vi "Lines GetSessionByName.vi"(8 "error in (no error)":errorcluster, 10 "[] Session Name":string, 11 "Config Text List":string[](array[string])=["[Datalog_Path]", "datalog_name_rule_1={Customer_ID}/{Device_Name}/{Customer_LotNo}/{Sub_LotNo}/", "datalog_name_rule_2={Subcon}_{Tester_ID}_{Mode_Code}_{Device_Name}_{Program_Name}_{Customer_LotNo}_{Sub_LotNo}_{Test_BinNo}_{Test_Code}_{End_Time}", "[Datalog_Type]", "edl_flag = false", "stdf_flag = true", "gdf_flag = true", "summary_flag = true", "txt_flag = true", "stdfconvert_flag = true", "[PackTestResult]", "PackTestResult = true", "PackFileType = gz", "PackFileSet = S", "[INPUT_OI_tester_id]", "Name = Tester_ID", "Pattern = ^[A-Z]|[0-9]+\\S*$", "Index = 0", "[INPUT_OI_operator_id]", "Name = Operator_ID", "Pattern = ^[A-Z]|[0-9]+\\S*$", "Index = 1", "[INPUT_OI_device_name]", "Name = Device_Name", "Pattern = ^[A-Z]|[0-9]+\\S*$", "Index = 2", "[INPUT_OI_lot_no]", "Name = Customer_LotNo", "Pattern = ^[A-Z]|[0-9]+\\S*$", "Index = 3", "[INPUT_OI_sublot]", "Name = Sub_LotNo", "Pattern = ^[A-Z]+[0-9]+\\S*$", "Index = 4", "[INPUT_OI_mode_code]", "Name = Mode_Code", "Pattern = ^FT1$", "Index = 5", "[INPUT_OI_test_code]", "Name = Test_Code", "Pattern = ^R\\d+(\\.\\d+)?$", "Index = 6", "[INPUT_OI_test_bin_no]", "Name = Test_BinNo", "Pattern = ^ALL$", "Index = 7", "[TestCode_Config]", "R0=P1", "R0.1=P2", "R0.2=P3", "R0.3=P4", "R0.4=P5", "R0.5=P6", "R0.6=P7", "R0.7=P8", "R1=R1", "R1.1=R1.1", "R1.2=R1.2", "R2=R2", "R2.1=R2.1", "R2.2=R2.2", "R3=R3", "R3.1=R3.1", "R3.2=R3.2", "R4=R4", "R4.1=R4.1", "R4.2=R4.2", "R5=R5", "R5.1=R5.1", "R5.2=R5.2", "R6=R6", "R6.1=R6.1", "R6.2=R6.2", "Q0=Q0", "Q0.1=Q0.1", "Q1=Q1", "Q2=Q2", "Q3=Q3", "Q4=Q4", "Q5=Q5", "Q6=Q6", "Q7=Q7", "[Stdf_variable_Config]", "Mode_Code=TEST_COD", "Test_Code=FLOW_ID", "[Stdf_constant_Config]", "JCET=FACIL_ID", "25C=TST_TEMP", "[special Control Flag]", "tester_check_flag = 0", "application_mode_flag = 0", "exec_input_flag = 0", "databridge_flag = 0", "[efuse check condition]", "efuse_check_flag = 0", "T8980+T9980=T9900或S8980+S9980=S9900或H8980+H9980=H9900（具体要看每个产品以什么方式体现）", "T9980<10", "[HardBin_Pass]", "PASS_BIN=1,2", "[HardBin_alarm]", "1<95%", "2>0.5%", "[HardBin_Define]", "1=PASS", "2=openshort", "3=functionfail", "4=functionfail", "5=functionfail", "6=functionfail", "8=functionfail", "[SoftBin_Pass]", "PASS_BIN=101,102", "[SoftBin_alarm]", "201>0.5%", "301>0.2%", "[SoftBin_Define]", "1=PASS_CLASS1", "101=RC_PASS", "200=OS_DPS_Short_failed_200", "220=OS_Func_VSS_RPT1_failed_220", "221=OS_PPMU_VSS_failed_221", "310=DC_VIH_VDDH_failed_310", "311=DC_VIL_VDDL_failed_311", "312=DC_IIHL_failed_312", "330=DC_VOHL_failed_330", "340=FC_IOZ_Func_failed_340", "341=DC_IOZ_failed_341", "370=DC_IDDDQ_Func_failed_370", "371=DC_IDDDQ_failed_371", "400=FC_BSCAN_failed_400", "410=FC_MBIST_RAM_SLOW_failed_410", "411=FC_MBIST_ROM_BASIC_failed_411", "412=FC_MBIST_SLOW_INCR1_failed_412", "413=FC_MBIST_SLOW_INCR2_failed_413", "414=FC_MBIST_CPU_ALL_failed_414", "415=FC_MBIST_FEPHY_failed_415", "416=FC_MBIST_ROM_FEPHY_failed_416", "420=FC_CHAIN_LOW_failed_420", "430=FC_STUCK_LOW_R02_1_430", "431=FC_STUCK_LOW_R02_1_431", "432=FC_STUCK_LOW_R02_2_432", "433=FC_STUCK_LOW_R02_3_433", "434=FC_STUCK_LOW_R02_4_434", "435=FC_STUCK_LOW_R02_5_435", "436=FC_STUCK_LOW_R02_6_436", "437=FC_STUCK_LOW_R02_7_437", "440=FC_TRANS_LOW_R02_failed_440", "441=FC_TRANS_LOW_1_failed_441", "442=FC_TRANS_LOW_2_failed_442", "443=FC_TRANS_LOW_3_failed_443", "444=FC_TRANS_LOW_4_failed_444", "445=FC_TRANS_LOW_5_failed_445", "446=FC_TRANS_LOW_6_failed_446", "447=FC_TRANS_LOW_7_failed_447", "448=FC_TRANS_LOW_8_failed_448", "449=FC_TRANS_LOW_9_failed_449", "450=FC_TRANS_LOW_10_failed_450", "451=FC_TRANS_LOW_11_failed_451", "452=FC_TRANS_LOW_12_failed_452", "453=FC_TRANS_LOW_13_failed_453", "454=FC_TRANS_LOW_14_failed_454", "455=FC_TRANS_LOW_15_failed_455", "456=FC_TRANS_LOW_16_failed_456", "457=FC_TRANS_LOW_17_failed_457", "458=FC_TRANS_LOW_18_failed_458", "460=FC_TRANS_LOW_GPU_1_failed_460", "461=FC_TRANS_LOW_GPU_2_failed_461", "462=FC_TRANS_LOW_GPU_3_failed_462", "463=FC_TRANS_LOW_GPU_4_failed_463", "464=FC_TRANS_LOW_GPU_5_failed_464", "465=FC_TRANS_LOW_GPU_6_failed_465", "471=FC_TRANS_LOW_CPU_1_failed_471", "472=FC_TRANS_LOW_CPU_2_failed_472", "473=FC_TRANS_LOW_CPU_3_failed_473", "480=FC_TRANS_LOW_GPU_failed_480", "490=FC_TRANS_LOW_CPU_failed_490", "500=FC_MBIST_CPU_ALL_GB_failed_500", "501=FC_MBIST_CPU_ALL_0P94_GB_failed_501", "510=BIST_USB3_EXTLP_0P95_GB_failed_510", "511=BIST_USB3_INTLP_0P95_GB_failed_511", "520=BIST_USB3_ASYNC_failed_520", "600=BIST_DDR_AC_failed_600", "601=BIST_DDR_DAT_INT_601", "602=BIST_DDR_AC_EXT_R15_failed_602", "603=BIST_DDR_DAT_EXT_R15_failed_603", "610=BIST_USB2_1P_FS_failed_610", "611=BIST_USB2_1P_HS_failed_611", "612=BIST_USB2_2P_FS_failed_612", "613=BIST_USB2_2P_HS_failed_613", "614=BIST_USB3_EXTLP_failed_614", "615=BIST_USB3_INTLP_failed_615", "620=BIST_PLL_failed_620", "630=FEPHY_CONFIG_failed_630", "631=FESTA220_MDIO_W_TEST_failed_631", "632=FESTA220_CD_RISE_failed_632", "633=FESTA220_CLK_BIST_failed_633", "634=Bin0634", "635=Bin0635", "636=FESTA220_RAMP_BIST_failed_636", "637=FESTA220_DO_ALL_AFE_BIST_failed_637", "638=FESTA220_AEQ_BIST_failed_638", "639=FESTA220_ATN_BIST_failed_639", "640=FESTA220_CD_STEP_BIST_failed_640", "641=FESTA220_ADCO_BIST_failed_641", "650=LDO_failed_650", "660=MX_ADAC_DYN_failed_660", "670=MX_VDAC_Static_failed_670", "671=MX_VDAC_Dynamic_failed_671", "680=HDMI_BIST_01_failed_680", "681=HDMI_BIST_02_failed_681", "682=HDMI_BIST_03_failed_682", "683=HDMI_BIST_04_failed_683", "684=HDMI_BIST_05_failed_684", "690=FC_Tsensor_failed_690", "800=OTP_BLANKTEST_failed_800", "801=OTP_TESTDEC_failed_801", "802=OTP_BLANKPRM_failed_802", "803=OTP_DOLBY_DISABLE_failed_803", "804=OTP_DOLBY_LOCK_failed_804", "805=OTP_DTS_ENABLE_failed_805", "806=OTP_DTS_LOCK_failed_806", "807=OTP_MV_EN_failed_807", "808=OTP_SOCFUSE_BGA19_failed_808", "809=OTP_DIEID_LOCK_failed_809", "812=OTP_SOCFUSE_LOCK_failed_812", "813=OTP_ATE_LOCK_failed_813", "814=OTP_LOTINFO_failed_814", "815=OTP_vendor_judge_failed_814", "816=OTP_ID_WORD_LOCK_failed_816", "820=OTP_TSENSOR_PGM_Failed_820", "821=OTP_TSENSOR_OTC_failed_821", "830=2OTP_TSENSOR_FRC_failed_822", "837=OTP_STA_Verimatrix_std_failed_837", "838=OTP_DYNAMIC_Verimatrix_adv_failed_838", "839=OTP_STATIC_Verimatrix_adv_failed_839", "880=OTP_ReTest_failed_880"]) -> (0 "error out":errorcluster, 2 "Session":string[](array[string]), 3 "Config Text List out":string[](array[string]))   [LabVIEW 2017, in "ini_configuration.lvlib"]
uses:
  ini_configuration.lvlib
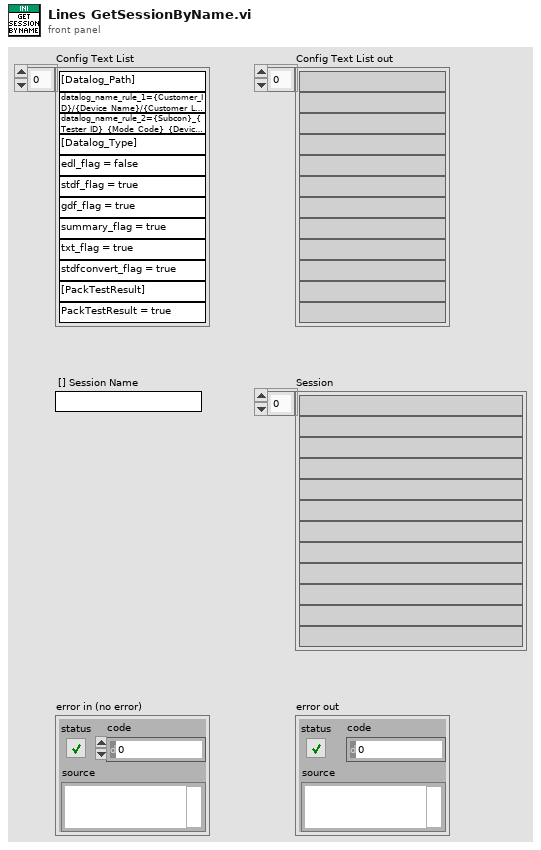
[diagram p1: front panel]
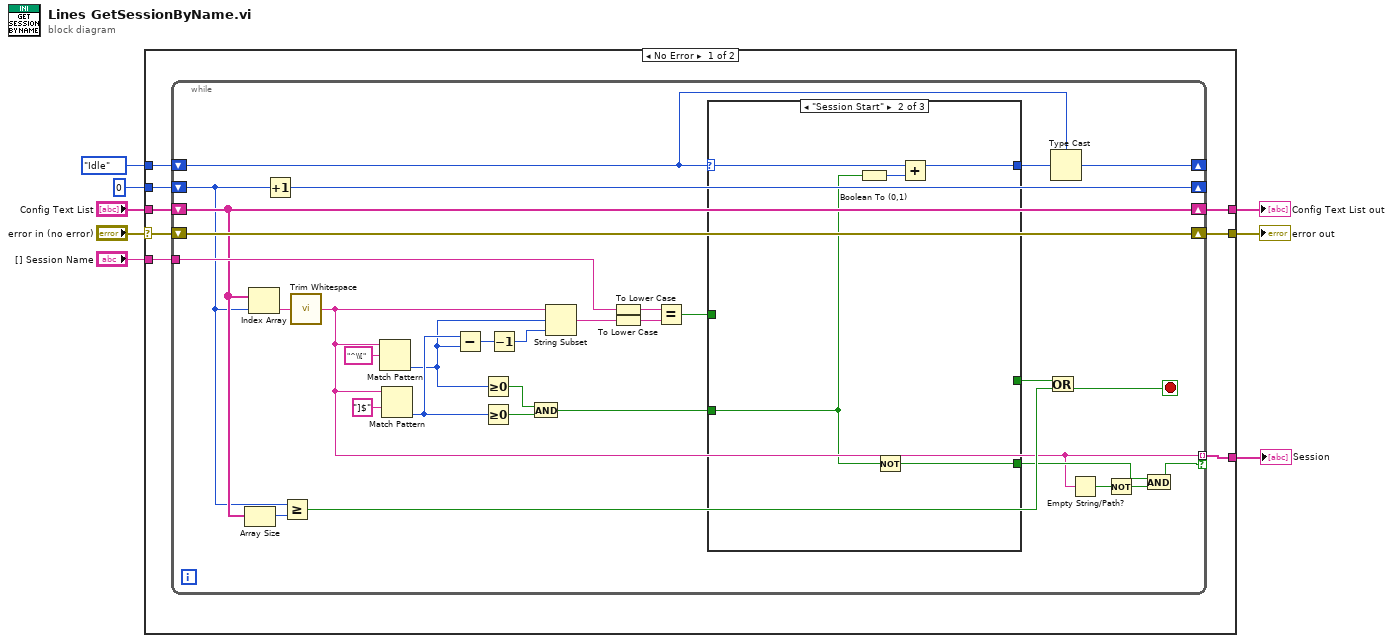
[diagram p0: block diagram]
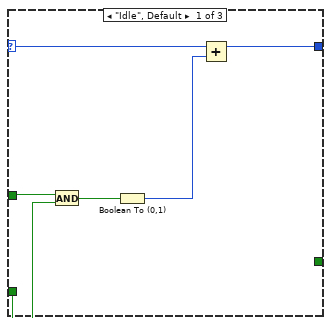
[diagram p2: hidden frame]
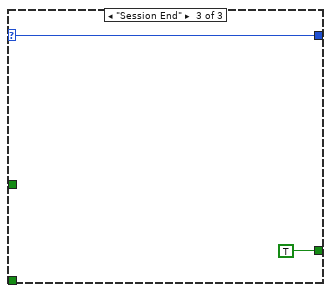
[diagram p3: hidden frame]
diagram:
  n1 = case shown="No Error" "error in (no error)" {
    selector: "error in (no error)" -> [w16 w62]
    tunnel: [w15 w62] -> w7
    tunnel: [w14 w61] -> w6
    tunnel: "Config Text List" -> [w13 w61]
    tunnel: 0 ("index(-1)") -> [w12 _]
    tunnel: "[] Session Name" -> [w11 _]
    tunnel: enum16{"Idle", "Session Start", "Session End"}."Idle" -> [w10 _]
    tunnel: [w9 _] -> w1
    frame No Error {
      n2 = while {
        shift-right: [w47] -> w15
        shift-left: w16 -> [w47]
        shift-right: [w31] -> w14
        shift-left: w13 -> [w31]
        shift-right: [w39] -> _
        shift-left: w12 -> [w29]
        tunnel: w11 -> [w37]
        shift-right: [w33] -> _
        shift-left: w10 -> [w32]
        tunnel: [w21] -> w9 mode=indexing if=w23
        stop <- w27 stop-if-true
        n3 = Array Size(array=w31) -> (size(s)=w30:i32)
        n4 = Index Array(array=w31, index=w29) -> (element=w24:string)
        n5 = Increment(x=w29) -> (x+1=w39:i32)
        n6 = Greater Or Equal?(x=w29, y=w30) -> (x >= y?=w28:bool)
        n7 = call <vilib>:"Trim Whitespace.vi"("string"=w24) -> ("trimmed string"=w21:string)  [unwired: 1 in]
        n8 = Match Pattern(string=w21, regular expression="^\\[") -> (offset past match=w42:i32)  [unwired: 1 in, 3 out]
        n9 = Match Pattern(string=w21, regular expression="]$") -> (offset past match=w43:i32)  [unwired: 1 in, 3 out]
        n10 = Subtract(x=w43, y=w42) -> (x-y=w41:i32)
        n11 = Greater Or Equal To 0?(x=w42) -> (x >= 0?=w45:bool)
        n12 = Greater Or Equal To 0?(x=w43) -> (x >= 0?=w44:bool)
        n13 = Decrement(x=w41) -> (x-1=w40:i32)
        n14 = And(x=w45, y=w44) -> (x .and. y?=w34:bool)
        n15 = String Subset(string=w21, offset (0)=w42, length (rest)=w40) -> (substring=w38:string)
        n16 = To Lower Case(string=w37) -> (all lower case string=w18:string)
        n17 = To Lower Case(string=w38) -> (all lower case string=w17:string)
        n18 = Equal?(x=w18, y=w17) -> (x = y?=w35:bool)
        n19 = case shown="\"Session Start\"" w32 {
          selector: w32 -> [w50 w57 w60]
          tunnel: [w53 w58 w60] -> w36
          tunnel: w35 -> [w52 _ _]
          tunnel: w34 -> [w51 w54 _]
          tunnel: [_ _ TRUE] -> w26
          tunnel: [_ w55 _] -> w22
          frame "Idle", Default {
            n20 = And(x=w52, y=w51) -> (x .and. y?=w49:bool)
            n21 = Boolean To (0,1)(Boolean=w49) -> (0, 1=w48:i16)
            n22 = Add(x=w50, y=w48) -> (x+y=w53:u16)
          }
          frame "Session Start" {
            n23 = Boolean To (0,1)(Boolean=w54) -> (0, 1=w56:i16)
            n24 = Not(x=w54) -> (.not. x?=w55:bool)
            n25 = Add(x=w57, y=w56) -> (x+y=w58:u16)
          }
          frame "Session End" {
          }
        }
        n26 = Or(x=w26, y=w28) -> (x .or. y?=w27:bool)
        n27 = Type Cast(type=w32, x=w36) -> (*(type *) &x=w33:enum16{"Idle", "Session Start", "Session End"})
        n28 = Empty String/Path?(string/path=w21) -> (empty?=w20:bool)
        n29 = Not(x=w20) -> (.not. x?=w19:bool)
        n30 = And(x=w22, y=w19) -> (x .and. y?=w23:bool)
      }
    }
    frame Error {
    }
  }
  "error out" <- w7
  "Config Text List out" <- w6
  "Session" <- w1
